vi "Begin.vi"(8 "error in":errorcluster) -> (0 "error out":errorcluster)   [LabVIEW 2018]
doc: "Called before other user functions, this VI is expected to open initial I/O refnums, load in file data, and do all program initialization. Notice that the <B>error out</B> terminal is simply used for data flow. Wiring it to other structures or subVIs ensures that this VI runs first."
uses:
  <userlib>/836-Library/System/TDMS_V2/Support/Logging_Settings.ctl
  <vilib>/Rock Robotics/WPI/DriverStation/WPI_DriverStationRobotMode2.ctl
  <vilib>/Rock Robotics/WPI/ThirdParty/Phoenix-LabVIEW/Motor Controller/Controls/CTRE_Phoenix_MotorControl_NeutralMode.ctl
  <vilib>/Rock Robotics/WPI/Solenoid/WPI_SolenoidChannel.ctl
  <vilib>/Rock Robotics/WPI/Joystick/WPI_JoystickDeviceEnum.ctl
  <vilib>/Rock Robotics/WPI/ThirdParty/Phoenix-LabVIEW/Motor Controller/Controls/CTRE_Phoenix_MotorControl_StatusFrameEnhanced.ctl
  <vilib>/Rock Robotics/WPI/ThirdParty/Phoenix-LabVIEW/Motor Controller/Controls/CTRE_Phoenix_MotorControl_FeedbackDevice.ctl
  <vilib>/Rock Robotics/WPI/ThirdParty/Phoenix-LabVIEW/Pigeon IMU/CTRE_PigeonIMU_StatusFrameRate.ctl
  Robot Global Data.vi
  <vilib>/Rock Robotics/WPI/ThirdParty/Phoenix-LabVIEW/Pigeon IMU/CTRE_PigeonIMU_Open_TalonSRX.vi
  <vilib>/Rock Robotics/WPI/Solenoid/WPI_SolenoidOpenSingle.vi
  <vilib>/Rock Robotics/WPI/Utilities/WPI_GetSetVariantRefNum.vi
  <userlib>/836-Library/System/TDMS_V2/Support/Channel_Config.ctl
  <userlib>/836-Library/System/TDMS_V2/Support/Group_Config.ctl
panel:
  in  "Logging Settings":T1={"Data Grab Period"=35.0, "File Write Period"=1000.0, "Max Stored Size"=100.0, "Burst Size"=150.0}
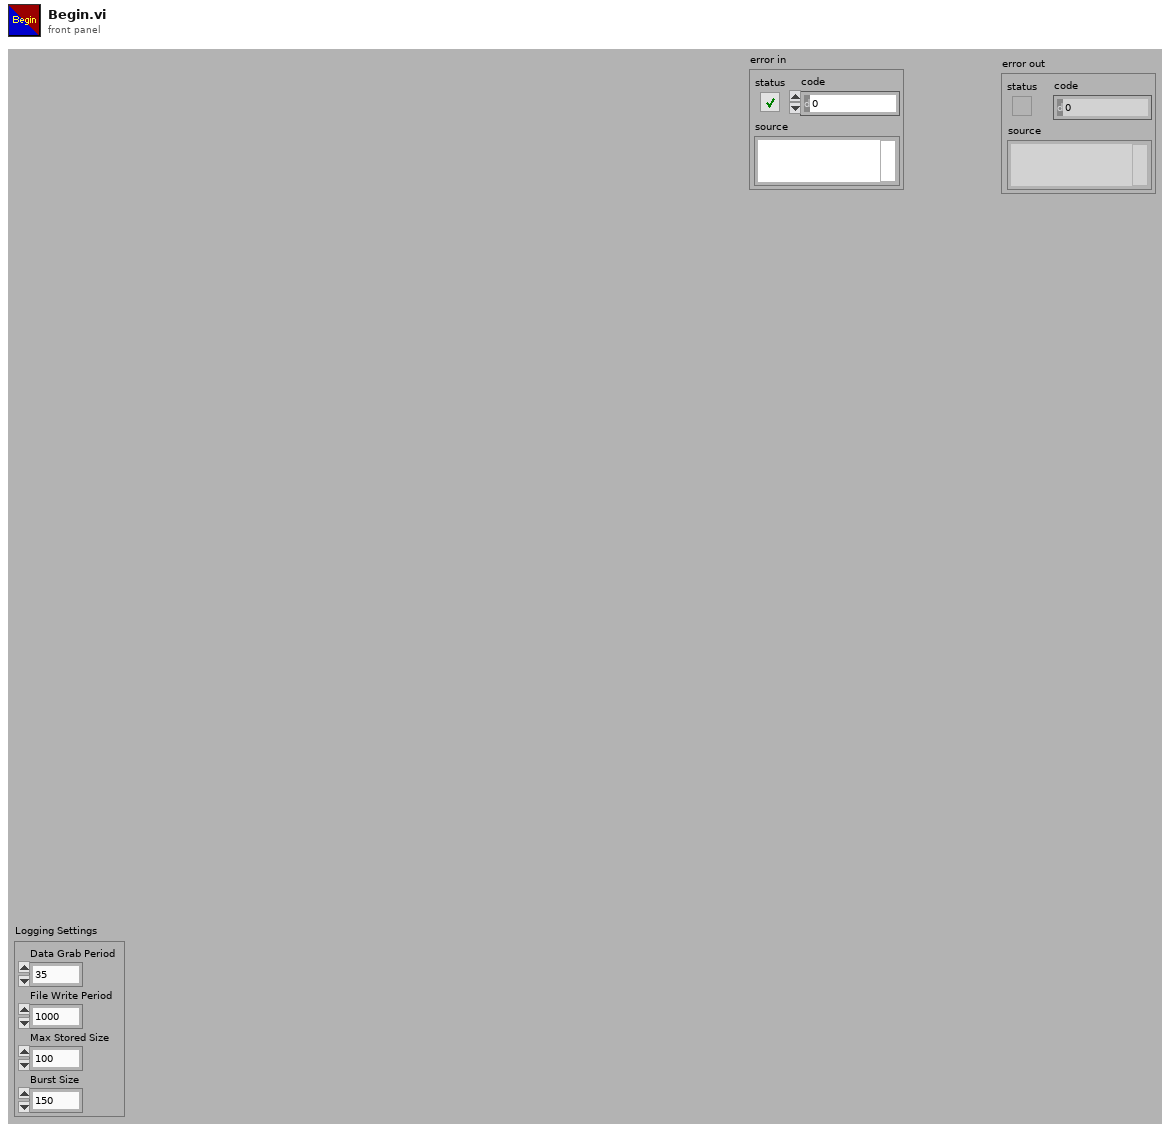
[diagram p1: front panel]
types:
  T1 = typedef "Logging_Settings.ctl" = cluster{"Data Grab Period":dbl, "File Write Period":dbl, "Max Stored Size":dbl, "Burst Size":dbl}
  T2 = typedef "CTRE_PigeonIMU_StatusFrameRate.ctl" = u32
  T3 = typedef "CTRE_Phoenix_MotorControl_FeedbackDevice.ctl" = i8
  T4 = typedef "CTRE_Phoenix_MotorControl_StatusFrameEnhanced.ctl" = u16
  T5 = typedef "WPI_SolenoidChannel.ctl" = enum8{"Solenoid 0", "Solenoid 1", "Solenoid 2", "Solenoid 3", "Solenoid 4", "Solenoid 5", "Solenoid 6", "Solenoid 7", "Invalid"}
  T6 = typedef "WPI_JoystickDeviceEnum.ctl" = enum16{"USB 0", "USB 1", "USB 2", "USB 3", "USB 4", "USB 5"}
  T7 = typedef "CTRE_Phoenix_MotorControl_NeutralMode.ctl" = enum8{"EEPROMSetting", "Override to Coast", "Override to Brake"}
  T8 = typedef "WPI_DriverStationRobotMode2.ctl" = enum16{"Autonomous Disabled", "Autonomous Enabled", "Teleop Disabled", "Teleop Enabled", "Disconnected", "Finish", "Test Disabled", "Test Enabled", "Emergency Stopped"}
  T9 = enum16{"open", "replace", "create", "open or create", "replace or create", "replace or create with confirmation"}
  T10 = typedef "Group_Config.ctl" = cluster{"Name":string, "Channel Config":T11}
  T11 = typedef "Channel_Config.ctl" = cluster{"Channel Names":string[]}
  T12 = typedef "WPI_CompressorDevRef.ctl" = cluster{"DevStatus":errorcluster, "Pneumatics Control Module":u8}
  T13 = typedef "WPI_JoystickDevRef.ctl" = cluster{"Device":T6}
  T14 = typedef "WPI_SolenoidDevRef.ctl" = cluster{"DevStatus":errorcluster, "Pneumatics Control Module":u8, "Forward Solenoid Channel":T5, "Reverse Solenoid Channel":T5}
  T15 = typedef "WPI_MotorControlDeviceRef.ctl" = cluster{"DeviceStatus":errorcluster, "Type":T16, "PWM":cluster{"PWM Channel":T17, "DeadBand":T18}, "CAN":cluster{"Device Number":u8, "SetOutput VI Ref":variant, "GetOutput VI Ref":variant, "Enable VI Ref":variant, "Disable VI Ref":variant, "Data":variant}, "Invert":bool, "DIO PWM":cluster{"PWM \"Enable\" Channel":T17, "DIOChannel":T19, "PWM Rate":dbl}}
  T16 = typedef "WPI_MotorControlType.ctl" = enum16{"PWM", "CAN", "DIO PWM"}
  T17 = typedef "FPGA_DIOPWMChannel.ctl" = enum8{"PWM 0", "PWM 1", "PWM 2", "PWM 3", "PWM 4", "PWM 5", "PWM 6", "PWM 7", "PWM 8", "PWM 9", "PWM MXP 0", "PWM MXP 1", "PWM MXP 2", "PWM MXP 3", "PWM MXP 4", "PWM MXP 5", "PWM MXP 6", "PWM MXP 7", "PWM MXP 8", "PWM MXP 9", "Invalid"}
  T18 = typedef "WPI_PWMDeadband.ctl" = cluster{"Name":string, "maxPositivePwm":i32, "minPositivePwm":i32, "centerPwm":i32, "maxNegativePwm":i32, "minNegativePwm":i32, "angularRange":u16}
  T19 = typedef "FPGA_DIOChannel.ctl" = enum8{"DIO 0", "DIO 1", "DIO 2", "DIO 3", "DIO 4", "DIO 5", "DIO 6", "DIO 7", "DIO 8", "DIO 9", "DIO MXP 0", "DIO MXP 1", "DIO MXP 2", "DIO MXP 3", "DIO MXP 4", "DIO MXP 5", "DIO MXP 6", "DIO MXP 7", "DIO MXP 8", "DIO MXP 9", "DIO MXP 10", "DIO MXP 11", "DIO MXP 12", "DIO MXP 13", "DIO MXP 14", "DIO MXP 15", "SPI Port CS1", "SPI Port CS2", "SPI Port CS3", "SPI Port MISO", "SPI Port MOSI", "Invalid"}
  T20 = typedef "CTRE_PigeonIMU_DeviceRef.ctl" = cluster{"DeviceStatus":errorcluster, "Device Number":u8, "Type":T21, "Device ID":u32, "Handle":u64, "UsageFrame":u32, "Library Path":path}
  T21 = typedef "CTRE_PigeonIMU_ConnectionType.ctl" = u32
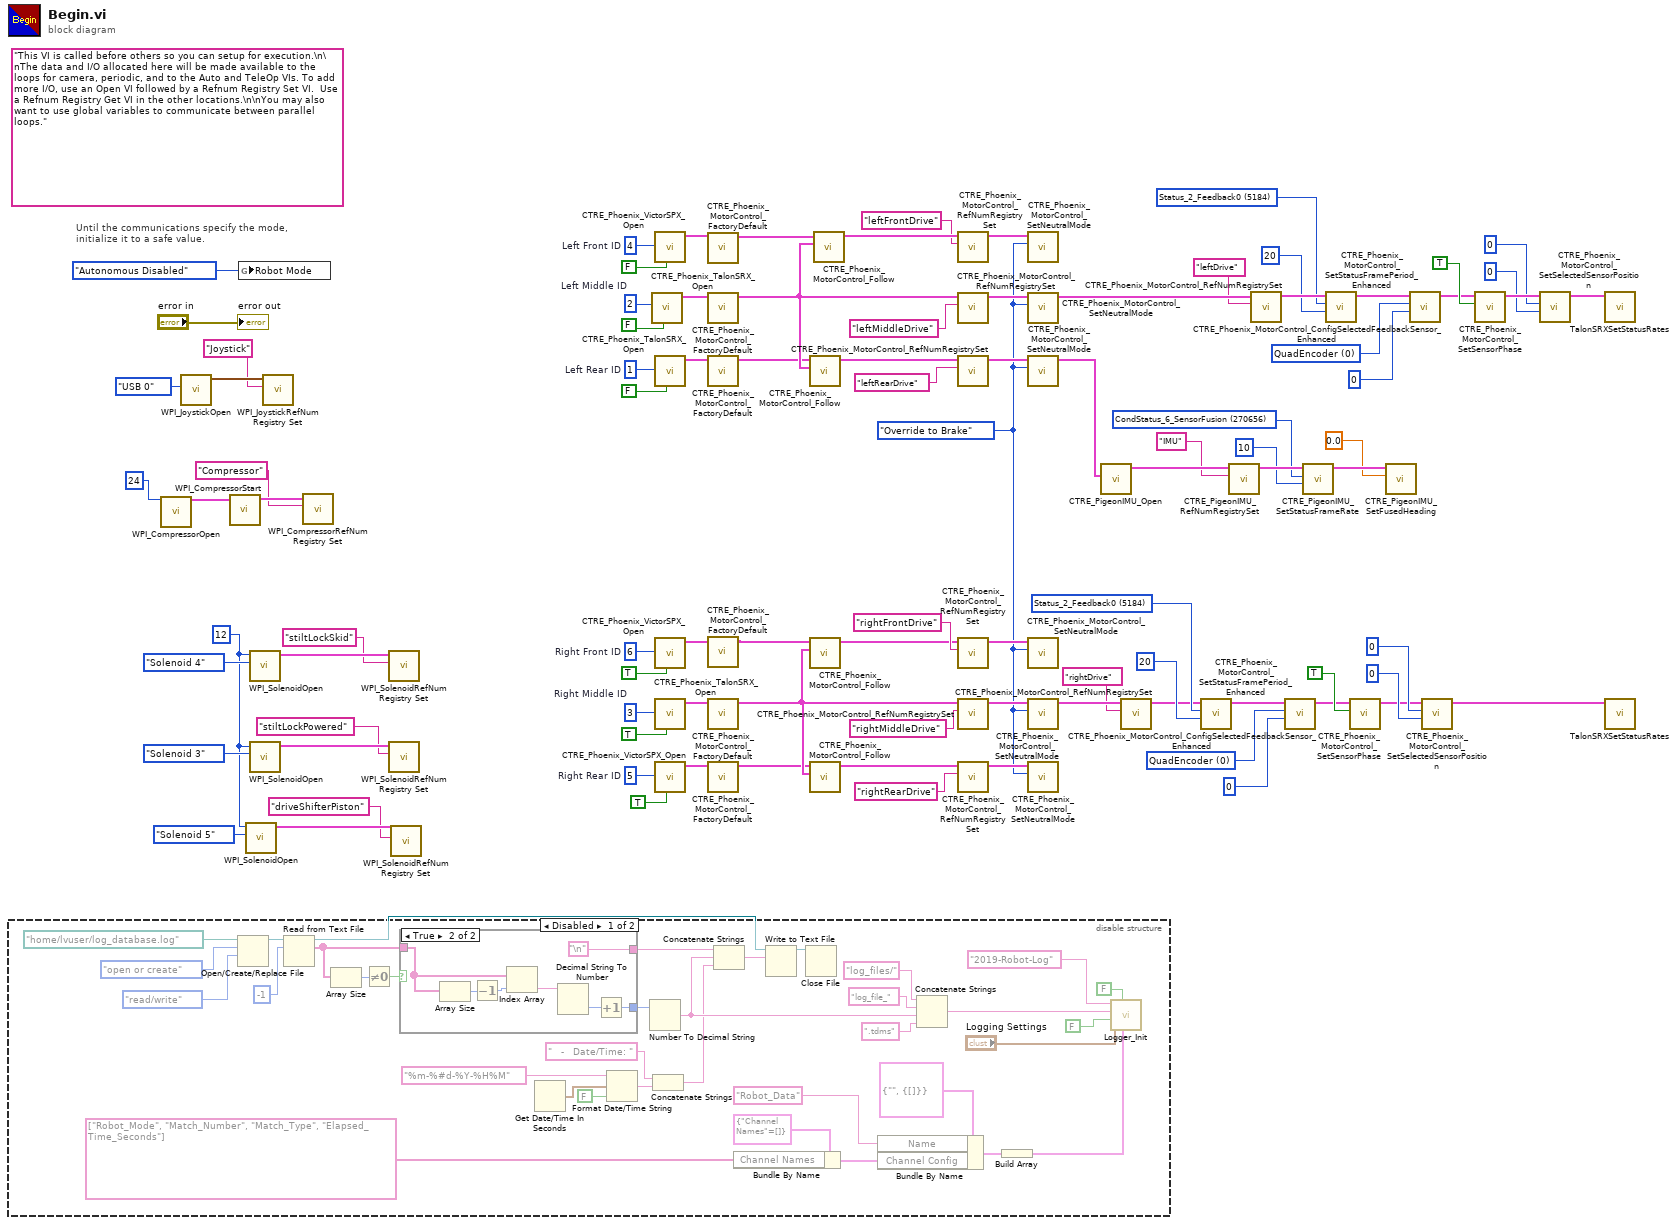
[diagram p0: block diagram]
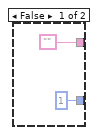
[diagram p2: hidden frame]
diagram:
  w12 = T2 270656 items=["CondStatus_1_General"=270336, "CondStatus_9_SixDeg_YPR"=270848, "CondStatus_6_SensorFusion"=270656, "CondStatus_11_GyroAccum"=270976, "CondStatus_2_GeneralCompass"=270400, "CondStatus_3_GeneralAccel"=270464, "CondStatus_10_SixDeg_Quat"=270912, "RawStatus_4_Mag"=265408, "BiasedStatus_2_Gyro"=269376, "BiasedStatus_4_Mag"=269504, "BiasedStatus_6_Accel"=269632] ("StatusFrame")
  w21 = T3 0 items=["QuadEncoder"=0, "Analog"=2, "Tachometer"=4, "Pulse Width Encoded Position"=8, "Sensor Sum (S0 + S1)"=9, "Sensor Difference (D0 - D1)"=10, "Remote Source 0"=11, "Remote Source 1"=12, "Software Emulated"=15] ("Feedback Device")
  w24 = T3 0 items=["QuadEncoder"=0, "Analog"=2, "Tachometer"=4, "Pulse Width Encoded Position"=8, "Sensor Sum (S0 + S1)"=9, "Sensor Difference (D0 - D1)"=10, "Remote Source 0"=11, "Remote Source 1"=12, "Software Emulated"=15] ("Feedback Device")
  w28 = T4 5184 items=["Status_1_General"=5120, "Status_2_Feedback0"=5184, "Status_3_Quadrature"=5248, "Status_4_AinTempVbat"=5312, "Status_6_Misc"=5440, "Status_7_CommStatus"=5504, "Status_8_PulseWidth"=5568, "Status_9_MotProfBuffer"=5632, "Status_10_MotionMagic"=5696, "Status_11_UartGadgeteer"=5760, "Status_12_Feedback1"=5824, "Status_13_Base_PIDF0"=5888, "Status_14_Turn_PIDF1"=5952, "Status_15_FirmwareApiStatus"=6016] ("Status Frame")
  w31 = T4 5184 items=["Status_1_General"=5120, "Status_2_Feedback0"=5184, "Status_3_Quadrature"=5248, "Status_4_AinTempVbat"=5312, "Status_6_Misc"=5440, "Status_7_CommStatus"=5504, "Status_8_PulseWidth"=5568, "Status_9_MotProfBuffer"=5632, "Status_10_MotionMagic"=5696, "Status_11_UartGadgeteer"=5760, "Status_12_Feedback1"=5824, "Status_13_Base_PIDF0"=5888, "Status_14_Turn_PIDF1"=5952, "Status_15_FirmwareApiStatus"=6016] ("Status Frame")
  w47 = u8 12 ("Pneumatics Control Module (0)")
  w67 = CTRE_Phoenix_MotorControl_NeutralMode."Override to Brake" ("Motor Control Neutral Mode")
  w87 = u8 1  # Left Rear ID
  w79 = u8 2  # Left Middle ID
  w89 = u8 4  # Left Front ID
  w90 = u8 5  # Right Rear ID
  w92 = u8 3  # Right Middle ID
  w94 = u8 6  # Right Front ID
  (unwired) "This VI is called before others so you can setup for execution.\n\nThe data and I/O allocated here will be made available to the loops for camera, periodic, and to the Auto and TeleOp VIs. To add more I/O, use an Open VI followed by a Refnum Registry Set VI.  Use a Refnum Registry Get VI in the other locations.\n\nYou may also want to use global variables to communicate between parallel loops."
  # "Until the communications specify the mode,\ninitialize it to a safe value."
  n1 = disable-structure shown="Disabled" {
    frame Disabled {
      n2 = Open/Create/Replace File(file path (use dialog)=path "/home/lvuser/log_database.log", operation (0:open)=T9."open or create", access (0:read/write)=enum16{"read/write", "read-only", "write-only"}."read/write") -> (refnum out=w111:refnum<file>)  [unwired: 3 in, 2 out]
      n3 = Read from Text File(file (use dialog)=w111, count=-1) -> (refnum out=w104:refnum<file>, text=w110:string[])  [unwired: 2 in, 2 out]
      n4 = Array Size(array=w110) -> (size(s)=w108:i32)
      n5 = Not Equal To 0?(x=w108) -> (x != 0?=w109:bool)
      n6 = case shown="True" w109 {
        tunnel: [1 w139] -> w107
        tunnel: w110 -> [_ w138]
        tunnel: ["" "\n"] -> w106
        frame False {
        }
        frame True {
          n7 = Array Size(array=w138) -> (size(s)=w137:i32)
          n8 = Decrement(x=w137) -> (x-1=w136:i32)
          n9 = Index Array(array=w138, index=w136) -> (element=w135:string)
          n10 = Decimal String To Number(string=w135) -> (number=w140:i32)  [unwired: 2 in, 1 out]
          n11 = Increment(x=w140) -> (x+1=w139:i32)
        }
      }
      n12 = Get Date/Time In Seconds() -> (seconds since 1Jan1904=w100:timestamp)
      n13 = Format Date/Time String(time format string (%c)="%m-%#d-%Y-%H%M", seconds (now)=w100, UTC format=FALSE) -> (date/time string=w98:string)
      n14 = Number To Decimal String(number=w107) -> (decimal integer string=w103:string)  [unwired: 1 in]
      n15 = Concatenate Strings("   -   Date/Time: " ("string"), w98) -> (w99:string)
      n16 = Concatenate Strings(w106, w103, w99) -> (w105:string)
      n17 = Bundle By Name(cluster=T11 {"Channel Names"=[]} ("Channel Config"), "Channel Names"=string[] ["Robot_Mode", "Match_Number", "Match_Type", "Elapsed_Time_Seconds"]) -> (w122:T11)
      n18 = Write to Text File(file (use dialog)=w104, text=w105) -> (refnum out=w112:refnum<file>)  [unwired: 2 in, 2 out]
      n19 = Close File(refnum=w112) -> ()  [unwired: 1 in, 2 out]
      n20 = Bundle By Name(cluster=T10 {"Name"="", "Channel Config"={"Channel Names"=[]}} ("Group Config"), "Name"="Robot_Data", "Channel Config"=w122) -> (w119:T10)
      n21 = Concatenate Strings("log_files/" ("string"), "log_file_" ("TDMS Name"), w103, ".tdms" ("string")) -> (w126:string)
      n22 = Build Array(w119) -> (w118:T10[])
      n23 = call <userlib>:"Logger_Init.vi"("Group Config"=w118, "Log To Computer?"=FALSE, "Logging Settings"="Logging Settings", "Log To USB?"=FALSE, "File Name"=w126, "Logger Name"="2019-Robot-Log") -> ()  [unwired: 4 in, 2 out]
    }
    frame Enabled {
    }
  }
  n24 = call <vilib>:"WPI_CompressorOpen.vi"("Pneumatics Control Module (0)"=u8 24) -> ("CompressorDevRef"=w59:T12)  [unwired: 13 in, 1 out]
  n25 = call <vilib>:"WPI_JoystickOpen.vi"("JoystickDevice"=WPI_JoystickDeviceEnum."USB 0") -> ("JoystickDevRef"=w55:T13)  [unwired: 10 in]
  n26 = call <vilib>:"WPI_CompressorStart.vi"("CompressorDevRef"=w59) -> ("CompressorDevRef"=w58:T12)  [unwired: 9 in, 1 out]
  n27 = global write "Robot Global Data.vi" "Robot Mode"(WPI_DriverStationRobotMode2."Autonomous Disabled" ("Robot Mode")) -> ()
  n28 = call-poly <vilib>:"WPI_SolenoidOpen.vi"("Solenoid Channel"=WPI_SolenoidChannel."Solenoid 5", "Pneumatics Control Module (0)"=w47) -> ("SolenoidDevRef"=w48:T14)  [unwired: 8 in, 1 out]
  n29 = call-poly <vilib>:"WPI_SolenoidOpen.vi"("Solenoid Channel"=WPI_SolenoidChannel."Solenoid 4", "Pneumatics Control Module (0)"=w47) -> ("SolenoidDevRef"=w65:T14)  [unwired: 8 in, 1 out]
  n30 = call-poly <vilib>:"WPI_SolenoidOpen.vi"("Solenoid Channel"=WPI_SolenoidChannel."Solenoid 3", "Pneumatics Control Module (0)"=w47) -> ("SolenoidDevRef"=w63:T14)  [unwired: 8 in, 1 out]
  n31 = call <vilib>:"WPI_JoystickRefNum Registry Set.vi"("refnum name"="Joystick", "JoystickDevRef"=w55) -> ()  [unwired: 8 in, 2 out]
  n32 = call <vilib>:"WPI_CompressorRefNum Registry Set.vi"("refnum name"="Compressor", "CompressorDevRef"=w58) -> ()  [unwired: 8 in, 2 out]
  n33 = call <vilib>:"WPI_SolenoidRefNum Registry Set.vi"("refnum name"="stiltLockSkid", "SolenoidDevRef"=w65) -> ()  [unwired: 8 in, 2 out]
  n34 = call <vilib>:"WPI_SolenoidRefNum Registry Set.vi"("refnum name"="stiltLockPowered", "SolenoidDevRef"=w63) -> ()  [unwired: 8 in, 2 out]
  n35 = call <vilib>:"WPI_SolenoidRefNum Registry Set.vi"("refnum name"="driveShifterPiston", "SolenoidDevRef"=w48) -> ()  [unwired: 8 in, 2 out]
  n36 = call <vilib>:"CTRE_Phoenix_TalonSRX_Open.vi"("Invert"=FALSE, "Device Number"=w79) -> ("CAN Talon SRX Ref"=w44:T15)  [unwired: 8 in, 1 out]
  n37 = call <vilib>:"CTRE_Phoenix_VictorSPX_Open.vi"("Invert"=FALSE, "Device Number"=w89) -> ("CAN Talon SRX Ref"=w34:T15)  [unwired: 8 in, 1 out]
  n38 = call <vilib>:"CTRE_Phoenix_TalonSRX_Open.vi"("Invert"=FALSE, "Device Number"=w87) -> ("CAN Talon SRX Ref"=w36:T15)  [unwired: 8 in, 1 out]
  n39 = call <vilib>:"CTRE_Phoenix_VictorSPX_Open.vi"("Invert"=TRUE, "Device Number"=w94) -> ("CAN Talon SRX Ref"=w42:T15)  [unwired: 8 in, 1 out]
  n40 = call <vilib>:"CTRE_Phoenix_TalonSRX_Open.vi"("Invert"=TRUE, "Device Number"=w92) -> ("CAN Talon SRX Ref"=w40:T15)  [unwired: 8 in, 1 out]
  n41 = call <vilib>:"CTRE_Phoenix_VictorSPX_Open.vi"("Invert"=TRUE, "Device Number"=w90) -> ("CAN Talon SRX Ref"=w38:T15)  [unwired: 8 in, 1 out]
  n42 = call <vilib>:"CTRE_Phoenix_MotorControl_FactoryDefault.vi"("PhoenixMotorControlDevRef"=w34) -> ("PhoenixMotorControlDevRef"=w33:T15)  [unwired: 9 in, 1 out]
  n43 = call <vilib>:"CTRE_Phoenix_MotorControl_FactoryDefault.vi"("PhoenixMotorControlDevRef"=w44) -> ("PhoenixMotorControlDevRef"=w43:T15)  [unwired: 9 in, 1 out]
  n44 = call <vilib>:"CTRE_Phoenix_MotorControl_FactoryDefault.vi"("PhoenixMotorControlDevRef"=w36) -> ("PhoenixMotorControlDevRef"=w35:T15)  [unwired: 9 in, 1 out]
  n45 = call <vilib>:"CTRE_Phoenix_MotorControl_FactoryDefault.vi"("PhoenixMotorControlDevRef"=w42) -> ("PhoenixMotorControlDevRef"=w41:T15)  [unwired: 9 in, 1 out]
  n46 = call <vilib>:"CTRE_Phoenix_MotorControl_FactoryDefault.vi"("PhoenixMotorControlDevRef"=w40) -> ("PhoenixMotorControlDevRef"=w39:T15)  [unwired: 9 in, 1 out]
  n47 = call <vilib>:"CTRE_Phoenix_MotorControl_FactoryDefault.vi"("PhoenixMotorControlDevRef"=w38) -> ("PhoenixMotorControlDevRef"=w37:T15)  [unwired: 9 in, 1 out]
  n48 = call <vilib>:"CTRE_Phoenix_MotorControl_Follow.vi"("Master Controller to Follow"=w43, "PhoenixMotorControlDevRef"=w35) -> ("PhoenixMotorControlDevRef"=w85:T15)  [unwired: 8 in, 1 out]
  n49 = call <vilib>:"CTRE_Phoenix_MotorControl_Follow.vi"("Master Controller to Follow"=w39, "PhoenixMotorControlDevRef"=w41) -> ("PhoenixMotorControlDevRef"=w76:T15)  [unwired: 8 in, 1 out]
  n50 = call <vilib>:"CTRE_Phoenix_MotorControl_Follow.vi"("Master Controller to Follow"=w39, "PhoenixMotorControlDevRef"=w37) -> ("PhoenixMotorControlDevRef"=w84:T15)  [unwired: 8 in, 1 out]
  n51 = call <vilib>:"CTRE_Phoenix_MotorControl_Follow.vi"("Master Controller to Follow"=w43, "PhoenixMotorControlDevRef"=w33) -> ("PhoenixMotorControlDevRef"=w77:T15)  [unwired: 8 in, 1 out]
  n52 = call <vilib>:"CTRE_Phoenix_MotorControl_RefNumRegistrySet.vi"("refnum name"="leftFrontDrive", "PhoenixMotorControlDevRef"=w77) -> ("PhoenixMotorControlDevRef"=w73:T15)  [unwired: 8 in, 1 out]
  n53 = call <vilib>:"CTRE_Phoenix_MotorControl_RefNumRegistrySet.vi"("refnum name"="leftMiddleDrive", "PhoenixMotorControlDevRef"=w43) -> ("PhoenixMotorControlDevRef"=w72:T15)  [unwired: 8 in, 1 out]
  n54 = call <vilib>:"CTRE_Phoenix_MotorControl_RefNumRegistrySet.vi"("refnum name"="leftRearDrive", "PhoenixMotorControlDevRef"=w85) -> ("PhoenixMotorControlDevRef"=w71:T15)  [unwired: 8 in, 1 out]
  n55 = call <vilib>:"CTRE_Phoenix_MotorControl_RefNumRegistrySet.vi"("refnum name"="rightFrontDrive", "PhoenixMotorControlDevRef"=w76) -> ("PhoenixMotorControlDevRef"=w70:T15)  [unwired: 8 in, 1 out]
  n56 = call <vilib>:"CTRE_Phoenix_MotorControl_RefNumRegistrySet.vi"("refnum name"="rightMiddleDrive", "PhoenixMotorControlDevRef"=w39) -> ("PhoenixMotorControlDevRef"=w69:T15)  [unwired: 8 in, 1 out]
  n57 = call <vilib>:"CTRE_Phoenix_MotorControl_RefNumRegistrySet.vi"("refnum name"="rightRearDrive", "PhoenixMotorControlDevRef"=w84) -> ("PhoenixMotorControlDevRef"=w68:T15)  [unwired: 8 in, 1 out]
  n58 = call <vilib>:"CTRE_Phoenix_MotorControl_SetNeutralMode.vi"("Motor Control Neutral Mode"=w67, "PhoenixMotorControlDevRef"=w73) -> ()  [unwired: 8 in, 2 out]
  n59 = call <vilib>:"CTRE_Phoenix_MotorControl_SetNeutralMode.vi"("Motor Control Neutral Mode"=w67, "PhoenixMotorControlDevRef"=w72) -> ("PhoenixMotorControlDevRef"=w52:T15)  [unwired: 8 in, 1 out]
  n60 = call <vilib>:"CTRE_Phoenix_MotorControl_SetNeutralMode.vi"("Motor Control Neutral Mode"=w67, "PhoenixMotorControlDevRef"=w71) -> ("PhoenixMotorControlDevRef"=w16:T15)  [unwired: 8 in, 1 out]
  n61 = call <vilib>:"CTRE_Phoenix_MotorControl_SetNeutralMode.vi"("Motor Control Neutral Mode"=w67, "PhoenixMotorControlDevRef"=w70) -> ()  [unwired: 8 in, 2 out]
  n62 = call <vilib>:"CTRE_Phoenix_MotorControl_SetNeutralMode.vi"("Motor Control Neutral Mode"=w67, "PhoenixMotorControlDevRef"=w69) -> ("PhoenixMotorControlDevRef"=w51:T15)  [unwired: 8 in, 1 out]
  n63 = call <vilib>:"CTRE_Phoenix_MotorControl_SetNeutralMode.vi"("Motor Control Neutral Mode"=w67, "PhoenixMotorControlDevRef"=w68) -> ()  [unwired: 8 in, 2 out]
  n64 = call-poly <vilib>:"CTRE_PigeonIMU_Open.vi"("CAN Talon SRX Ref"=w16) -> ("PigeonIMUDevRef"=w15:T20)  [unwired: 9 in, 1 out]
  n65 = call <vilib>:"CTRE_Phoenix_MotorControl_RefNumRegistrySet.vi"("refnum name"="rightDrive", "PhoenixMotorControlDevRef"=w51) -> ("PhoenixMotorControlDevRef"=w27:T15)  [unwired: 8 in, 1 out]
  n66 = call <vilib>:"CTRE_Phoenix_MotorControl_SetStatusFramePeriod_Enhanced.vi"("periodMs"=20, "Status Frame"=w28, "PhoenixMotorControlDevRef"=w27) -> ("PhoenixMotorControlDevRef"=w20:T15)  [unwired: 7 in, 1 out]
  n67 = call <vilib>:"CTRE_PigeonIMU_RefNumRegistrySet.vi"("refnum name"="IMU", "PigeonIMUDevRef"=w15) -> ("PigeonIMUDevRef"=w13:T20)  [unwired: 8 in, 1 out]
  n68 = call <vilib>:"CTRE_Phoenix_MotorControl_RefNumRegistrySet.vi"("refnum name"="leftDrive", "PhoenixMotorControlDevRef"=w52) -> ("PhoenixMotorControlDevRef"=w32:T15)  [unwired: 8 in, 1 out]
  n69 = call <vilib>:"CTRE_Phoenix_MotorControl_ConfigSelectedFeedbackSensor_Enhanced.vi"("pidLoopIdx"=0, "Feedback Device"=w21, "PhoenixMotorControlDevRef"=w20) -> ("PhoenixMotorControlDevRef"=w19:T15)  [unwired: 7 in, 1 out]
  n70 = call <vilib>:"CTRE_PigeonIMU_SetStatusFrameRate.vi"("Period (ms)"=i16 10, "StatusFrame"=w12, "PigeonIMUDevRef"=w13) -> ("PigeonIMUDevRef"=w10:T20)  [unwired: 7 in, 1 out]
  n71 = call <vilib>:"CTRE_Phoenix_MotorControl_SetStatusFramePeriod_Enhanced.vi"("periodMs"=20, "Status Frame"=w31, "PhoenixMotorControlDevRef"=w32) -> ("PhoenixMotorControlDevRef"=w25:T15)  [unwired: 7 in, 1 out]
  n72 = call <vilib>:"CTRE_Phoenix_MotorControl_SetSensorPhase.vi"("PhaseSensor"=TRUE, "PhoenixMotorControlDevRef"=w19) -> ("PhoenixMotorControlDevRef"=w3:T15)  [unwired: 8 in, 1 out]
  n73 = call <vilib>:"CTRE_PigeonIMU_SetFusedHeading.vi"("Value"=0.0, "PigeonIMUDevRef 2"=w10) -> ()  [unwired: 8 in, 2 out]
  n74 = call <vilib>:"CTRE_Phoenix_MotorControl_ConfigSelectedFeedbackSensor_Enhanced.vi"("pidLoopIdx"=0, "Feedback Device"=w24, "PhoenixMotorControlDevRef"=w25) -> ("PhoenixMotorControlDevRef"=w17:T15)  [unwired: 7 in, 1 out]
  n75 = call <vilib>:"CTRE_Phoenix_MotorControl_SetSelectedSensorPosition.vi"("pidLoopIdx"=u32 0, "New Sensor Position"=0, "PhoenixMotorControlDevRef"=w3) -> ("PhoenixMotorControlDevRef"=w1:T15)  [unwired: 7 in, 1 out]
  n76 = call <vilib>:"CTRE_Phoenix_MotorControl_SetSensorPhase.vi"("PhaseSensor"=TRUE, "PhoenixMotorControlDevRef"=w17) -> ("PhoenixMotorControlDevRef"=w8:T15)  [unwired: 8 in, 1 out]
  n77 = call <vilib>:"CTRE_Phoenix_MotorControl_SetSelectedSensorPosition.vi"("pidLoopIdx"=u32 0, "New Sensor Position"=0, "PhoenixMotorControlDevRef"=w8) -> ("PhoenixMotorControlDevRef"=w2:T15)  [unwired: 7 in, 1 out]
  n78 = call "TalonSRXSetStatusRates.vi"("Talon SRX DevRef In"=w2) -> ()  [unwired: 10 in, 1 out]
  n79 = call "TalonSRXSetStatusRates.vi"("Talon SRX DevRef In"=w1) -> ()  [unwired: 10 in, 1 out]
  "error out" <- "error in"
